vi "ConvertSpectrumToXYGraph.vi"(4 "spectrum":cluster{"frequency":dbl, "amplitude":dbl}[](array[cluster])) -> (1 "xy graph":cluster{"frequency":dbl[], "amplitude":dbl[]})   [LabVIEW 2017, in "EmsaAnalysis.lvlib"]
uses:
  <vilib>/addons/InsightCM/Devices/Shared/Emsa/EmsaAnalysis/EmsaAnalysis.lvlib
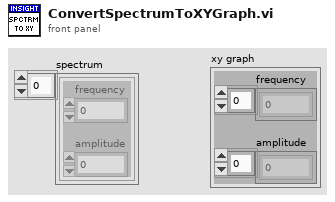
[diagram p1: front panel]
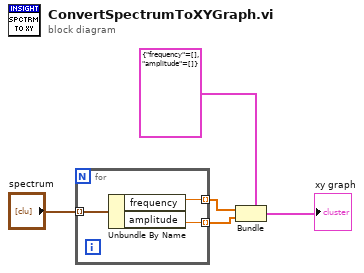
[diagram p0: block diagram]
diagram:
  n1 = for {
    tunnel: "spectrum" -> [w8] mode=indexing
    tunnel: [w7] -> w3 mode=indexing
    tunnel: [w6] -> w4 mode=indexing
    n2 = Unbundle By Name(w8) -> ("frequency"=w7:dbl, "amplitude"=w6:dbl)
  }
  n3 = Bundle(cluster=cluster{"frequency":dbl[], "amplitude":dbl[]} {"frequency"=[], "amplitude"=[]}, "frequency"=w3, "amplitude"=w4) -> (→"xy graph":cluster{"frequency":dbl[], "amplitude":dbl[]})
